vi "IsFirstIteration.vi"(1 "Left Hand":bool, 2 "AssessmentMode":T1, 3 "Trial Nr":i16) -> (0 "Is First Iteration":bool)   [LabVIEW 2015]
uses:
  All_In_One/States/Assessment_Modes.ctl
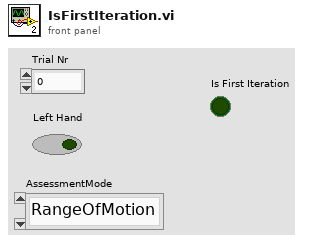
[diagram p1: front panel]
types:
  T1 = typedef "Assessment_Modes.ctl" = enum8{"RangeOfMotion", "Force", "Motor", "Sensorimotor", "PositionMatching", "PreciseReaching"}
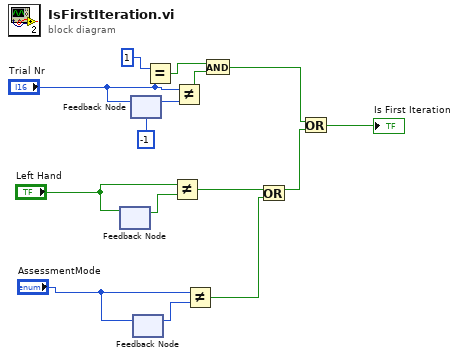
[diagram p0: block diagram]
diagram:
  n1 = feedback #1() -> (w9:bool)  [unwired: 1 in]
  n2 = feedback-in #1("Left Hand") -> ()
  n3 = feedback #2(i16 -1 ("Trial Nr")) -> (w15:i16)
  n4 = feedback-in #2("Trial Nr") -> ()
  n5 = feedback #3() -> (w4:T1)  [unwired: 1 in]
  n6 = feedback-in #3("AssessmentMode") -> ()
  n7 = Equal?(x=i16 1 ("y"), y="Trial Nr") -> (x = y?=w12:bool)
  n8 = Not Equal?(x="Left Hand", y=w9) -> (x != y?=w7:bool)
  n9 = Not Equal?(x="Trial Nr", y=w15) -> (x != y?=w13:bool)
  n10 = Not Equal?(x="AssessmentMode", y=w4) -> (x != y?=w1:bool)
  n11 = And(x=w12, y=w13) -> (x .and. y?=w6:bool)
  n12 = Or(x=w7, y=w1) -> (x .or. y?=w2:bool)
  n13 = Or(x=w6, y=w2) -> (x .or. y?=→"Is First Iteration":bool)
